vi "Set IPS Switch Heater.vi"(8 "error in (no error)":errorcluster, 10 "Switch Heater Status":T1, 11 "Instrument.Oxford1820 in":refnum<class "Instrument.Oxford1820.lvclass">) -> (0 "error out":errorcluster, 2 "Response":string, 3 "Instrument.Oxford1820 out":refnum<class "Instrument.Oxford1820.lvclass">)   [LabVIEW 2016, in "Instrument.Oxford1820.lvclass"]
uses:
  Instrument.Oxford1820.lvclass
  <instrlib>/Mercury iXX/Public/Libraries/Magnet/Controls/Switch Heater.ctl
  Instrument.Oxford1820.lvclass/Instrument.Oxford1820.ctl
  <instrlib>/Mercury iXX/Public/Libraries/Magnet/Open/Open Magnet Device.vi
  <instrlib>/Mercury iXX/Public/Libraries/Magnet/Signals/Set/Switch Heater Status (Set).vi
  <instrlib>/Mercury iXX/Public/Libraries/Magnet/Signals/Read/Switch Heater Status (Read).vi
  <instrlib>/Mercury iXX/Mercury iXX.lvlib
  <instrlib>/Mercury iXX/Public/Libraries/Magnet.lvlib
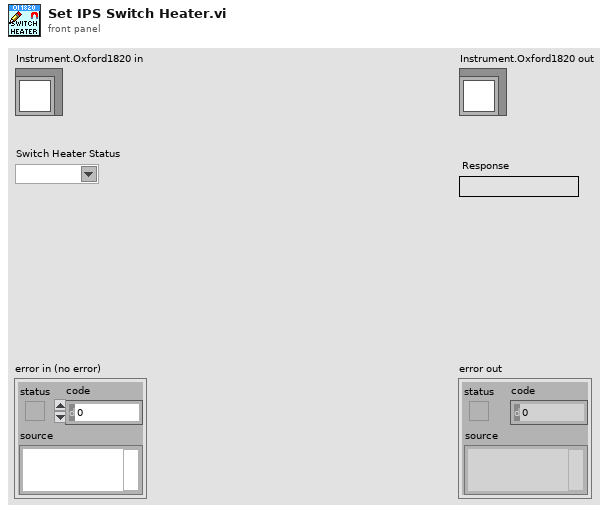
[diagram p1: front panel]
types:
  T1 = typedef "Mercury iXX.lvlib/Magnet.lvlib/Switch Heater.ctl" = string
  T2 = typedef "Mercury iXX.lvlib/Mercury Reference.ctl" = cluster{"Comms":refnum<visa-resource-name>, "Device ID":string[], "Comms Layer":T3, "Command":string, "Query reference":T4}
  T3 = typedef "Mercury iXX.lvlib/Comms Transport Layer.ctl" = enum16{"Ethernet TCP/IP", "USB", "ISOBus - RS-232", "GPIB"}
  T4 = typedef "Mercury iXX.lvlib/Query Dynamic Reference.ctl" = refnum<vi>
  T5 = typedef "Mercury iXX.lvlib/Response String.ctl" = string
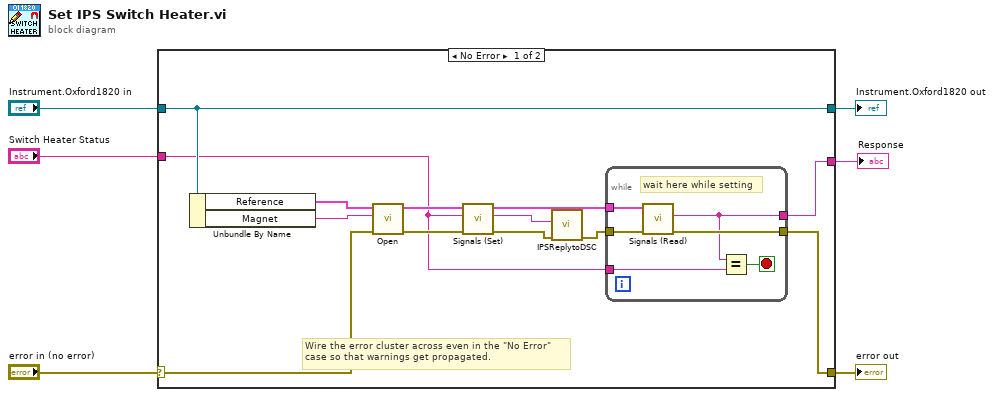
[diagram p0: block diagram]
diagram:
  n1 = case shown="No Error" "error in (no error)" {
    selector: "error in (no error)" -> [w16 w27]
    tunnel: [w9 w27] -> w5
    tunnel: [w19 w26] -> w3
    tunnel: "Instrument.Oxford1820 in" -> [w19 w26]
    tunnel: [w7 _] -> w2
    tunnel: "Switch Heater Status" -> [w11 _]
    frame No Error {
      # "Wire the error cluster across even in the \"No Error\"\ncase so that warnings get propagated."
      n2 = Unbundle By Name(w19) -> ("Reference"=w17:T2, "Magnet"=w18:string)
      n3 = call-poly <instrlib>:"Open.vi"("error in (no error)"=w16, "Device Identifier"=w18, "Mercury Reference In"=w17) -> ("error out"=w15:errorcluster, "Mercury Reference Out"=w14:T2)  [unwired: 7 out]
      n4 = call-poly <instrlib>:"Signals (Set).vi"("error in"=w15, "Switch Heater Status"=w11, "Mercury Reference In"=w14) -> ("error out"=w13:errorcluster, "Response"=w8:T5, "Mercury Reference Out"=w12:T2)  [unwired: 1 in, 5 out]
      n5 = call "IPSReplytoDSC.vi"("error in (no error)"=w13, "Response"=w8) -> ("error out"=w10:errorcluster)  [unwired: 9 in]
      n6 = while {
        tunnel: [w25] -> w9
        tunnel: w10 -> [w24]
        tunnel: w11 -> [w23]
        tunnel: w12 -> [w21]
        tunnel: [w20] -> w7
        stop <- w22 stop-if-true
        # "wait here while setting"
        n7 = call-poly <instrlib>:"Signals (Read).vi"("error in"=w24, "Mercury Reference In"=w21) -> ("error out"=w25:errorcluster, "Switch Heater Status"=w20:string)  [unwired: 1 in, 7 out]
        n8 = Equal?(x=w20, y=w23) -> (x = y?=w22:bool)
      }
    }
    frame Error {
    }
  }
  "error out" <- w5
  "Instrument.Oxford1820 out" <- w3
  "Response" <- w2
